vi "SCapture.vi"() -> ()   [LabVIEW 2019]
doc: "This VI captures the region of the screen and displays it on the front panel continuously.\nCan be used to develop remote desktop applications."
uses:
  <vilib>/Utility/miscctls.llb/LVBoundsTypeDef.ctl
  System.Drawing
  <vilib>/Utility/inputDevices.llb/mouseAcquire.vi
  <vilib>/Utility/inputDevices.llb/closeMouse.vi
  <vilib>/wsapi/NI_WebServices.lvlib
panel:
  out "Filtered String Output":string
  in  "Delay (ms)":i32=100
  in  "error in":errorcluster
  out "Mouse y":dbl
  out "Mouse x":dbl
  in  "Height (px)":i32=100
  in  "Width (px)":i32=100
  out "Screen Capture":picture
  in  "stop":bool
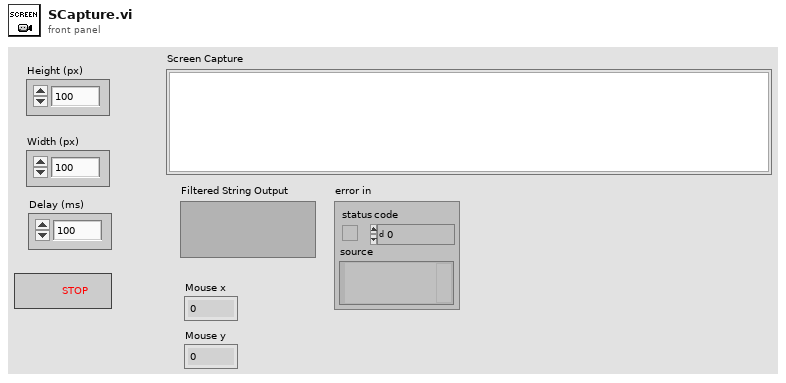
[diagram p1: front panel]
types:
  T1 = typedef "LVBoundsTypeDef.ctl" = cluster{"Width":u32, "Height":u32}
  T2 = typedef "Image Type" = u32
  T3 = cluster{"Horizontal":i32, "Vertical":i32, "Scrolling":i32}
  T4 = typedef "IMAQ Image.ctl" = refnum<image>
  T5 = typedef "imagedata.ctl" = cluster{"image type":i32, "image depth":i32, "image":u8[], "mask":u8[], "colors":u32[], "Rectangle":cluster{"left":i16, "top":i16, "right":i16, "bottom":i16}}
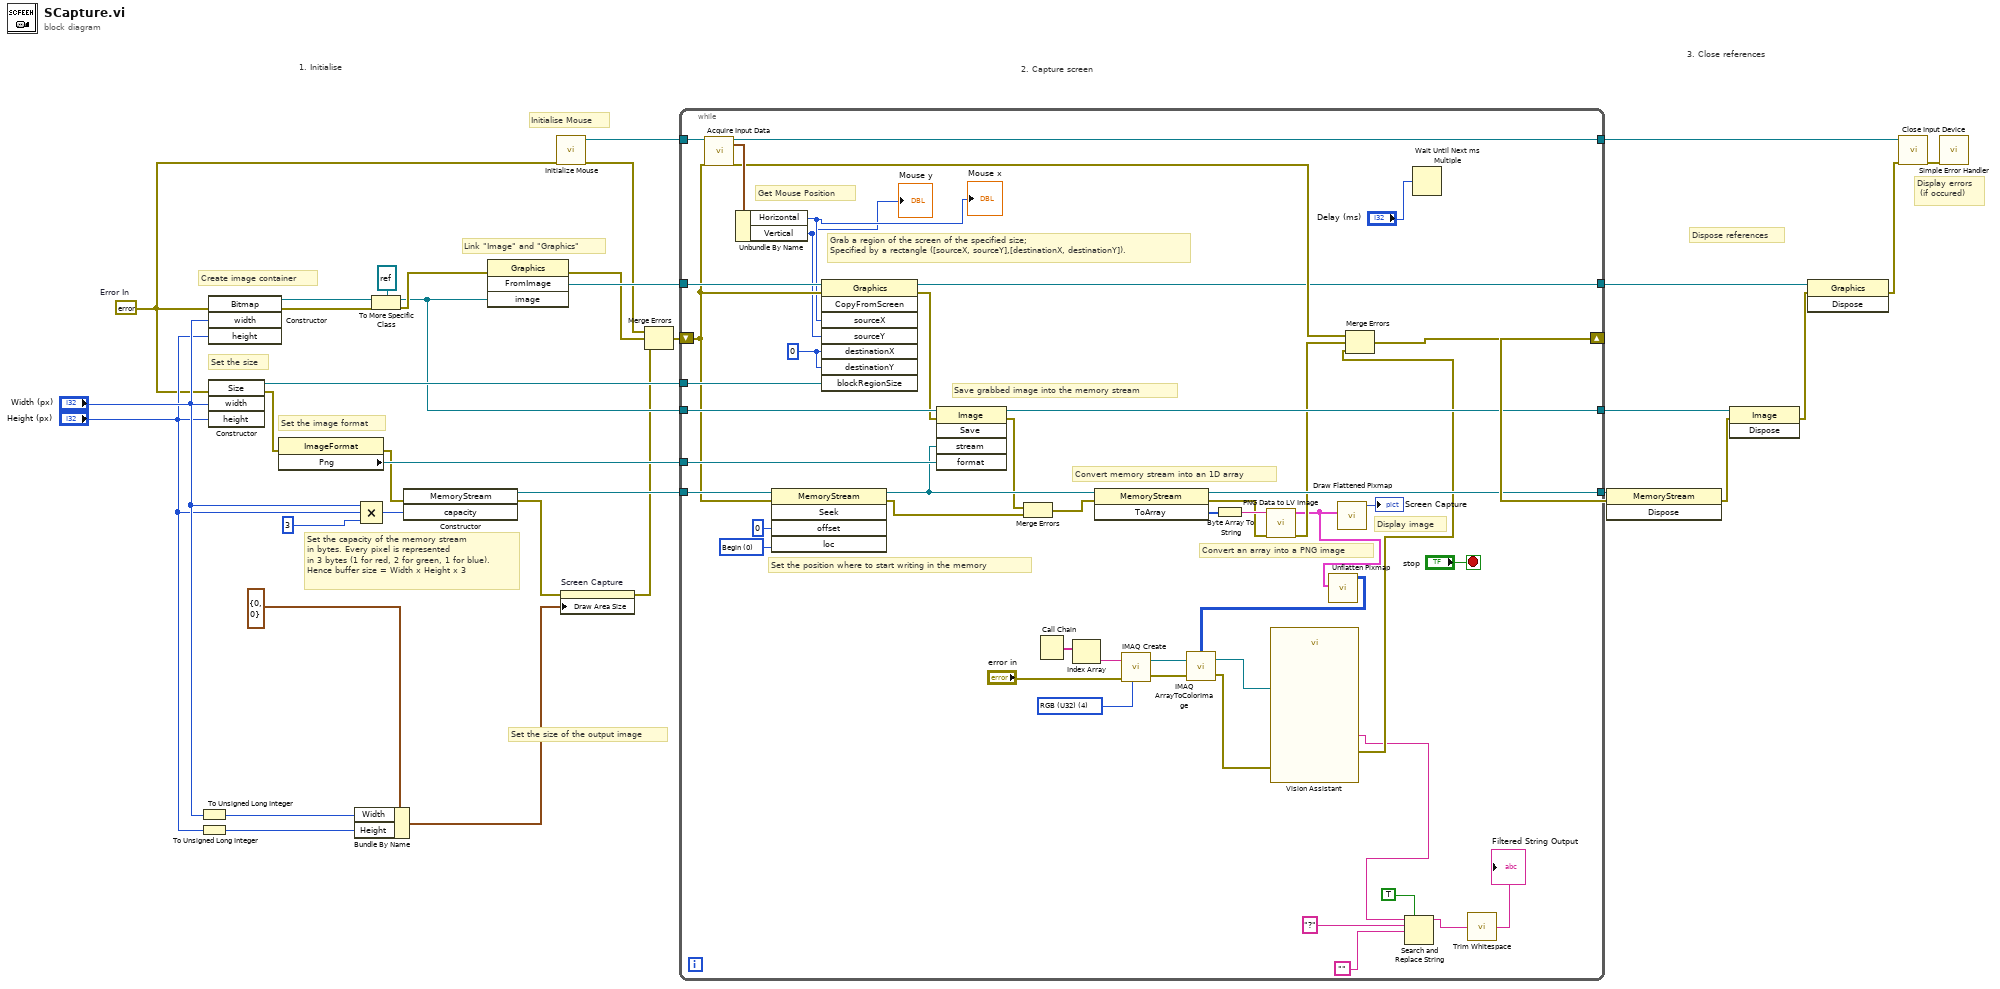
[diagram p0: block diagram]
diagram:
  w1 = errorcluster {"status"=FALSE, "code"=0, "source"=""}  # Error In
  # "Link \"Image\" and \"Graphics\""
  # "Set the size"
  # "Create image container"
  # "3. Close references"
  # "2. Capture screen"
  # "1. Initialise"
  # "Display errors\n (if occured)"
  # "Dispose references"
  # "Set the image format"
  # "Set the size of the output image"
  # "Set the capacity of the memory stream\nin bytes. Every pixel is represented\nin 3 bytes (1 for red, 2 for green, 1 for blue).\nHence buffer size = Width x Height x 3"
  # "Initialise Mouse"
  n1 = To Unsigned Long Integer(number="Width (px)") -> (unsigned 32bit integer=w9:u32)
  n2 = To Unsigned Long Integer(number="Height (px)") -> (unsigned 32bit integer=w7:u32)
  n3 = constructor class="Bitmap"(error in=w1, "width"="Width (px)", "height"="Height (px)") -> (reference out=w29:refnum<k24>, error out=w32:errorcluster)  [unwired: 2 in, 3 out]
  n4 = constructor class="Size"(error in=w1, "width"="Width (px)", "height"="Height (px)") -> (reference out=w27:refnum<k24>, error out=w18:errorcluster)  [unwired: 2 in, 3 out]
  n5 = property class="ImageFormat"(error in=w18) -> (error out=w17:errorcluster, "Png"=w26:refnum<k24>)  [unwired: 1 in, 1 out]
  n6 = Bundle By Name(cluster=T1 {"Width"=0, "Height"=0} ("Draw Area Size"), "Width"=w9, "Height"=w7) -> (w13:T1)
  n7 = Compound Arithmetic op=MULTIPLY("Width (px)", "Height (px)", 3 ("value")) -> (w21:i32)
  n8 = To More Specific Class(target class=refnum<k24> refnum, reference=w29, error in=w32) -> (specific class reference=w20:refnum<k24>, error out=w33:errorcluster)
  n9 = constructor class="MemoryStream"(error in=w17, "capacity"=w21) -> (reference out=w23:refnum<k24>, error out=w12:errorcluster)  [unwired: 2 in, 2 out]
  n10 = invoke class="Graphics" method="FromImage"(error in=w33, "image"=w20) -> (error out=w16:errorcluster, "FromImage"=w30:refnum<k24>)  [unwired: 2 in, 2 out]
  n11 = call <vilib>:"Initialize Mouse.vi"("error in (no error)"=w1) -> ("error out"=w14:errorcluster, "device ID"=w35:refnum<k1>)  [unwired: 9 in]
  n12 = property on="Screen Capture" class="Pict"(error in=w12, "Draw Area Size"=w13) -> (error out=w11:errorcluster)  [unwired: 1 in, 1 out]
  n13 = Merge Errors(w14, w16, w11) -> (w15:errorcluster)
  n14 = while {
    tunnel: w35 -> [w83]
    tunnel: [w81] -> w34
    tunnel: w30 -> [w80]
    tunnel: [w77] -> w28
    tunnel: w27 -> [w76]
    tunnel: w26 -> [w75]
    tunnel: [w74] -> w25
    tunnel: w23 -> [w73]
    tunnel: w20 -> [w66]
    shift-right: [w57] -> w6
    shift-left: w15 -> [w60]
    tunnel: [w56] -> w5
    stop <- "stop" stop-if-true
    w48 = T2 4 items=["Grayscale (U8)", "Grayscale (I16)", "Grayscale (SGL)", "Complex (CSG)", "RGB (U32)", "HSL (U32)", "RGB (U64)", "Grayscale (U16)"] ("Image Type")
    w67 = 0 ("destinationX")
    w71 = 0 items=["Begin", "Current", "End"] ("loc")
    # "Display image"
    # "Convert an array into a PNG image"
    # "Set the position where to start writing in the memory"
    # "Convert memory stream into an 1D array"
    # "Save grabbed image into the memory stream"
    # "Grab a region of the screen of the specified size;\nSpecified by a rectangle ([sourceX, sourceY],[destinationX, destinationY])."
    # "Get Mouse Position"
    n15 = call-poly <vilib>:"Acquire Input Data.vi"("device ID"=w83, "error in (no error)"=w60) -> ("device ID"=w81:refnum<k1>, "axis info"=w82:T3, "error out"=w59:errorcluster)  [unwired: 14 in, 1 out]
    n16 = Unbundle By Name(w82) -> ("Horizontal"=w55:i32, "Vertical"=w54:i32)
    "Mouse x" <- w55
    "Mouse y" <- w54
    n17 = invoke class="MemoryStream" method="Seek"(reference=w73, error in=w60, "offset"=i64 0, "loc"=w71) -> (reference out=w68:refnum<k24>, error out=w63:errorcluster)  [unwired: 1 in, 3 out]
    n18 = invoke class="Graphics" method="CopyFromScreen"(reference=w80, error in=w60, "sourceX"=w55, "sourceY"=w54, "destinationX"=w67, "destinationY"=w67, "blockRegionSize"=w76) -> (reference out=w56:refnum<k24>, error out=w61:errorcluster)  [unwired: 1 in, 6 out]
    n19 = invoke class="Image" method="Save"(reference=w66, error in=w61, "stream"=w68, "format"=w75) -> (reference out=w74:refnum<k24>, error out=w64:errorcluster)  [unwired: 1 in, 3 out]
    n20 = Merge Errors(w64, w63) -> (w62:errorcluster)
    n21 = Call Chain() -> (call chain=w50:string[])
    n22 = Index Array(array=w50) -> (element=w51:string)  [unwired: 1 in]
    n23 = invoke class="MemoryStream" method="ToArray"(reference=w68, error in=w62) -> (reference out=w77:refnum<k24>, error out=w65:errorcluster, "ToArray"=w79:u8[])  [unwired: 1 in]
    n24 = call "IMAQ Create"("Image Name"=w51, "Image Type"=w48, "error in (no error)"="error in") -> ("New Image"=w47:T4, "error out"=w46:errorcluster)  [unwired: 1 in, 1 out]
    n25 = Byte Array To String(unsigned byte array=w79) -> (string=w78:string)
    n26 = call <vilib>:"PNG Data to LV Image.vi"("error in (no error)"=w65, "png data"=w78) -> ("error out"=w58:errorcluster, "image data"=w53:T5)  [unwired: 8 in]
    n27 = call <vilib>:"Unflatten Pixmap.vi"("image data"=w53) -> ("24-bit pixmap"=w52:u32[][])  [unwired: 4 in, 6 out]
    n28 = call "IMAQ ArrayToColorImage"("Image Pixels (U32)"=w52, "Image"=w47, "error in (no error)"=w46) -> ("Image Out"=w43:T4, "error out"=w45:errorcluster)  [unwired: 2 in]
    n29 = call "Vision Assistant"("Image In"=w43, "error in"=w45) -> ("String (OCR/OCV 2)"=w38:string, "error out"=w44:errorcluster)  [unwired: 23 in, 1 out]
    n30 = call <vilib>:"Draw Flattened Pixmap.vi"("image data"=w53) -> ("new picture"=→"Screen Capture":picture)  [unwired: 8 in]
    n31 = Merge Errors(w59, w58, w44) -> (w57:errorcluster)
    n32 = Search and Replace String(replace all?=TRUE ("replace all? (F)"), input string=w38, search string="?", replace string="") -> (result string=w37:string)  [unwired: 4 in, 3 out]
    n33 = Wait Until Next ms Multiple(millisecond multiple="Delay (ms)") -> ()  [unwired: 1 out]
    n34 = call <vilib>:"Trim Whitespace.vi"("string"=w37) -> ("trimmed string"=→"Filtered String Output":string)  [unwired: 1 in]
  }
  n35 = invoke class="MemoryStream" method="Dispose"(reference=w28, error in=w6) -> (error out=w24:errorcluster)  [unwired: 1 in, 2 out]
  n36 = invoke class="Image" method="Dispose"(reference=w25, error in=w24) -> (error out=w4:errorcluster)  [unwired: 1 in, 2 out]
  n37 = invoke class="Graphics" method="Dispose"(reference=w5, error in=w4) -> (error out=w3:errorcluster)  [unwired: 1 in, 2 out]
  n38 = call-poly <vilib>:"Close Input Device.vi"("error in (no error)"=w3, "device ID"=w34) -> ("error out"=w2:errorcluster)  [unwired: 8 in]
  n39 = call <vilib>:"Simple Error Handler.vi"("error in (no error)"=w2) -> ()  [unwired: 4 in, 5 out]
